vi "ErrorCheck.vi"(8 "error in (no error)":errorcluster, 11 "I2C Data in":u8[](array[numeric])) -> (0 "error out":errorcluster)   [LabVIEW 2015, in "navX Library v3.lvlib" / "navX - I2C.lvclass"]
uses:
  navX - I2C.lvclass
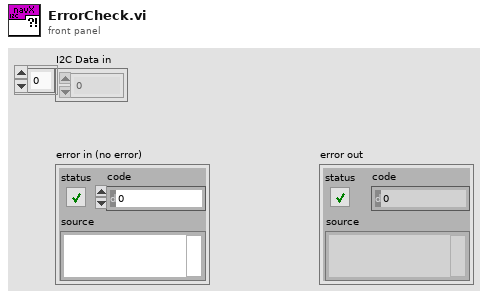
[diagram p1: front panel]
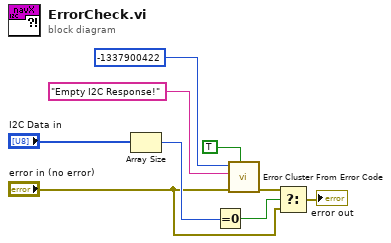
[diagram p0: block diagram]
diagram:
  n1 = Array Size(array="I2C Data in") -> (size(s)=w9:i32)
  n2 = Equal To 0?(x=w9) -> (x = 0?=w5:bool)
  n3 = call <vilib>:"Error Cluster From Error Code.vi"("show call chain? (False)"=TRUE, "error in (no error)"="error in (no error)", "error message (\"\")"="Empty I2C Response!" ("error message (\"\")"), "error code (0)"=-1337900422) -> ("error out"=w4:errorcluster)  [unwired: 5 in]
  n4 = Select(t=w4, s=w5, f="error in (no error)") -> (s? t:f=→"error out":errorcluster)
